vi "EMAPRE_REALTIME_VER2.0.vi"() -> ()   [LabVIEW 2015]
uses:
  <vilib>/Platform/TimedLoop/XDataNode/timing_clust.ctl
  <vilib>/Platform/TimedLoop/XDataNode/nitl_modes.ctl
  <vilib>/Platform/TimedLoop/XDataNode/wakeup.ctl
  <vilib>/myRIO/Common/Instrument Driver Framework/myRIO v1.0/AI/vis/myRIO v1.1 Open AI.vi
  <vilib>/myRIO/Common/Instrument Driver Framework/myRIO v1.0/UART/vis/myRIO v1.0 Close UART.vi
  <vilib>/myRIO/Common/Instrument Driver Framework/Utilities/vis/Validate Channels.vi
  <vilib>/myRIO/Common/Instrument Driver Framework/myRIO v1.0/AI/vis/myRIO v1.0 Reserve AI.vi
  <vilib>/myRIO/Common/Instrument Driver Framework/myRIO v1.0/AI/vis/myRIO v1.0 Build MUX Configuration AI.vi
  <vilib>/myRIO/Common/Instrument Driver Framework/myRIO v1.0/Resource Manager/vis/myRIO v1.0 Reserve Channel List.vi
  <vilib>/myRIO/Common/Instrument Driver Framework/myRIO v1.0/Resource Manager/vis/myRIO v1.0 Reserve Channel.vi
  <vilib>/myRIO/Common/Instrument Driver Framework/myRIO v1.0/Resource Manager/vis/myRIO v1.0 Unreserve Channel.vi
  <vilib>/myRIO/Common/Instrument Driver Framework/myRIO v1.0/Resource Manager/vis/myRIO v1.0 Build Mutex Name.vi
  <vilib>/Utility/VariantDataType/GetNumericInfo.vi
  <vilib>/Utility/error.llb/Error Cluster From Error Code.vi
  <vilib>/myRIO/Common/Instrument Driver Framework/myRIO v1.0/myRIO v1.1 Open.vi
  <vilib>/myRIO/Common/Instrument Driver Framework/myRIO v1.0/AI/vis/myRIO v1.0 Get Scaling Constants AI.vi
  <vilib>/myRIO/Common/Instrument Driver Framework/Utilities/vis/IO Manager.vi
  <vilib>/myRIO/Common/Instrument Driver Framework/Utilities/vis/Configuration Manager.vi
  <vilib>/myRIO/Common/Instrument Driver Framework/myRIO v1.0/myRIO v1.0 Close.vi
  <vilib>/myRIO/Common/Instrument Driver Framework/myRIO v1.0/AI/vis/myRIO v1.0 Read AI.vi
  <vilib>/myRIO/Common/Instrument Driver Framework/Utilities/vis/FPGA Ref Manager.vi
  <vilib>/myRIO/Common/Instrument Driver Framework/myRIO v1.0/myRIO v1.0 Reset FPGA.vi
  <vilib>/myRIO/Common/Instrument Driver Framework/myRIO v1.0/IRQ/vis/myRIO v1.0 IRQ Info FGV.vi
  <vilib>/myRIO/Common/Instrument Driver Framework/myRIO v1.0/IRQ/vis/myRIO v1.0 Timer IRQ Info FGV.vi
  <vilib>/myRIO/Common/Instrument Driver Framework/myRIO v1.0/IRQ/vis/myRIO v1.0 ISR Agent.vi
  <vilib>/platform/TimedLoop/XDataNode/XDataNode.xnode
  <vilib>/myRIO/Instrument Drivers/Onboard IO/AI/AI.lvlib
  <vilib>/myRIO/Instrument Drivers/Utilities/Utilities.lvlib
  <vilib>/Platform/TimedLoop/XDataNode/XDNodeRunTimeDep.lvlib
panel:
  in  "Body":string
  in  "Subject":string
  in  "Password":string
  in  "Email":string
  out "Time":timestamp format="%<%H:%M\n%d/%m/%y>T"
  out "Temperature":dbl(graph)
  out "Start Detection":bool
  in  "Current Sensor\nChannel":tag="B/AI0"
  in  "stop 2":bool
  out "Current Signal":dbl(graph)
  out "Fault":bool
  out "Good Condition":bool
  out "Temperature":dbl(slide) scale=0.0..100.0
  out "Temperature\n(Celcius)":dbl
  in  "stop":bool
  in  "Temperature Sensor\nChannel":tag="B/AI0"
  # "Stator Faults Detection on Induction Motor\n based on Electric Signals Measurement"
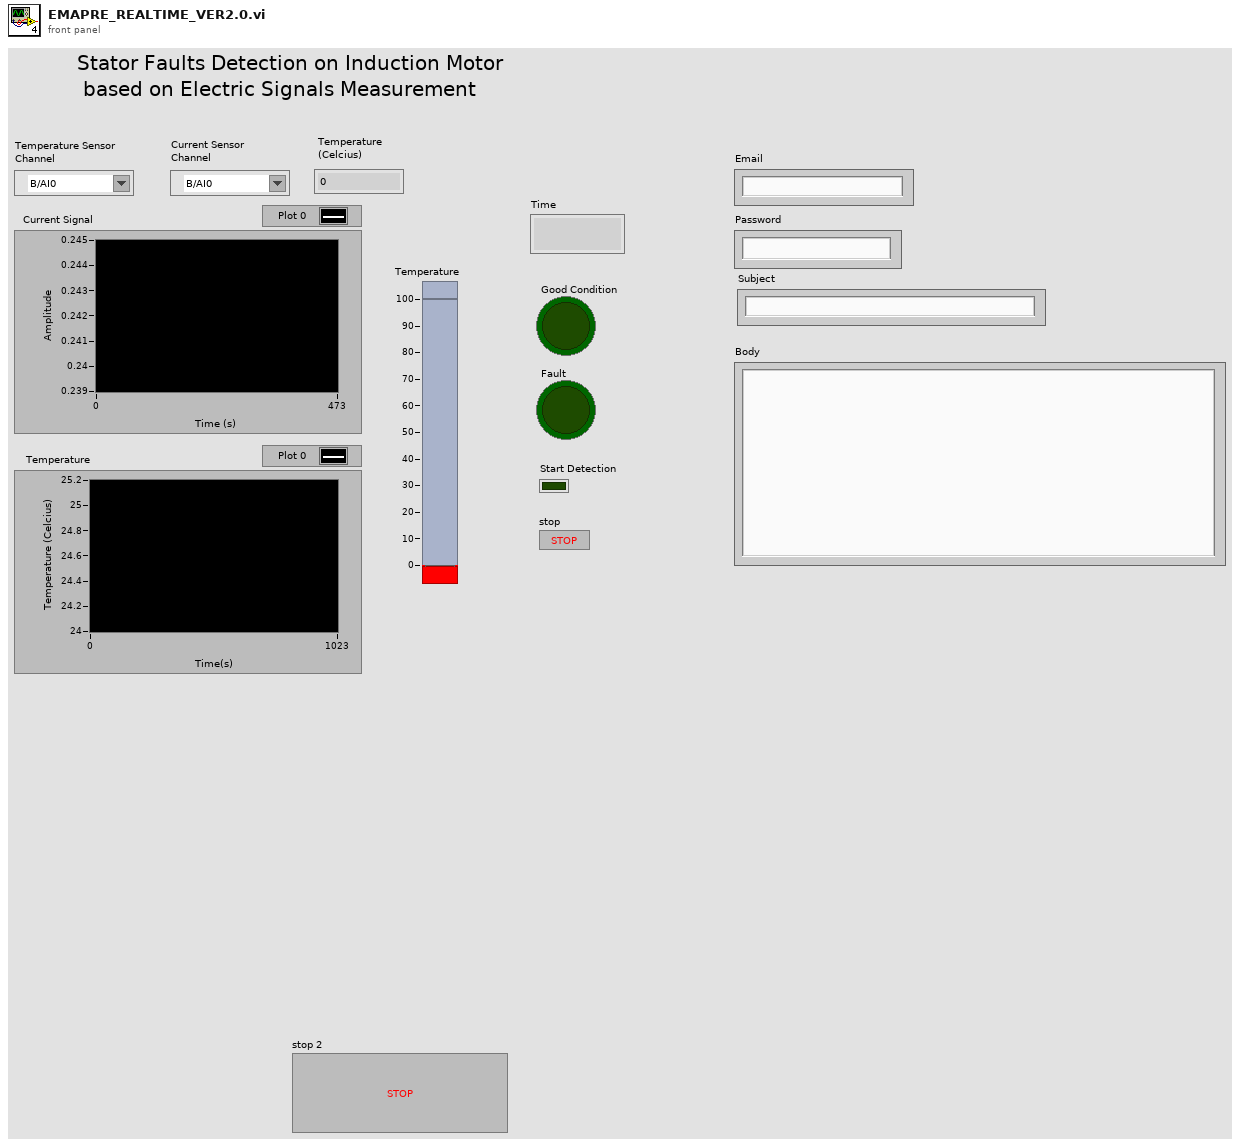
[diagram p1: front panel]
types:
  T1 = typedef "AI.lvlib/AI Reference.ctl" = cluster{"myRIO Reference":T2, "AI Channels List":T6, "AI Scaling Constants List":T8}
  T2 = typedef "myRIO Generic Hardware Reference.ctl" = cluster{"myRIO Model":T3, "myRIO Hardware Reference":T4}
  T3 = typedef "Hardware Version Enum.ctl" = enum16{"Unknown", "myRIO-1900", "myRIO-1950", "roboRIO"}
  T4 = typedef "myRIO v1.0 Reference.ctl" = cluster{"Generic FPGA Reference":T5, "Allow multiple opens":bool}
  T5 = typedef "Generic FPGA Reference.ctl" = refnum<k20>
  T6 = typedef "AI Channels List.ctl" = T7[]
  T7 = typedef "AI Channels Enum.ctl" = enum16{"Not Connected", "AudioIn/Left", "AudioIn/Right", "C/AI0", "C/AI1", "A/AI0", "A/AI1", "A/AI2", "A/AI3", "B/AI0", "B/AI1", "B/AI2", "B/AI3", "AI/AI0", "AI/AI1", "AI/AI2", "AI/AI3"}
  T8 = typedef "Analog Scaling Constants List.ctl" = T9[]
  T9 = typedef "Analog Scaling Constants.ctl" = cluster{"LSB Weight (Volts)":dbl, "Offset (Volts)":dbl, "Signed?":bool}
  T10 = typedef "XDNodeRunTimeDep.lvlib/timing_clust.ctl" = cluster{"Expected End [f-1]":u64, "Actual End [f-1]":u64, "Finished Late? [f-1]":bool, "Expected End [i-1]":u64, "Actual End [i-1]":u64, "Finished Late? [i-1]":bool, "Expected Start [i]":u64, "Actual Start [i]":u64, "Expected Start [f]":u64, "Actual Start [f]":u64, "Source Name":string, "Structure Name":string, "Period":i64, "Deadline":i64, "Offset":i64, "Start":i64, "Priority":i32, "Timeout":i32, "Mode":T11, "Wakeup Reason":T12, "Error":errorcluster, "Source Type":string, "Secondary Source Type":string, "Global End Time":u64, "Global Start Time":u64, "Frame Duration":u64, "Iteration Duration":u64, "Assigned CPU":i32, "I/O Scan Engine Mode":u32}
  T11 = typedef "XDNodeRunTimeDep.lvlib/nitl_modes.ctl" = enum32{"No Change", "Process missed periods, maintain original phase", "Discard missed periods, maintain original phase", "Process missed periods, ignore original phase", "Discard missed periods, ignore original phase"}
  T12 = typedef "XDNodeRunTimeDep.lvlib/wakeup.ctl" = enum32{"Normal", "Aborted", "Asynchronous wakeup", "Timing source error", "Timed loop error", "Timeout"}
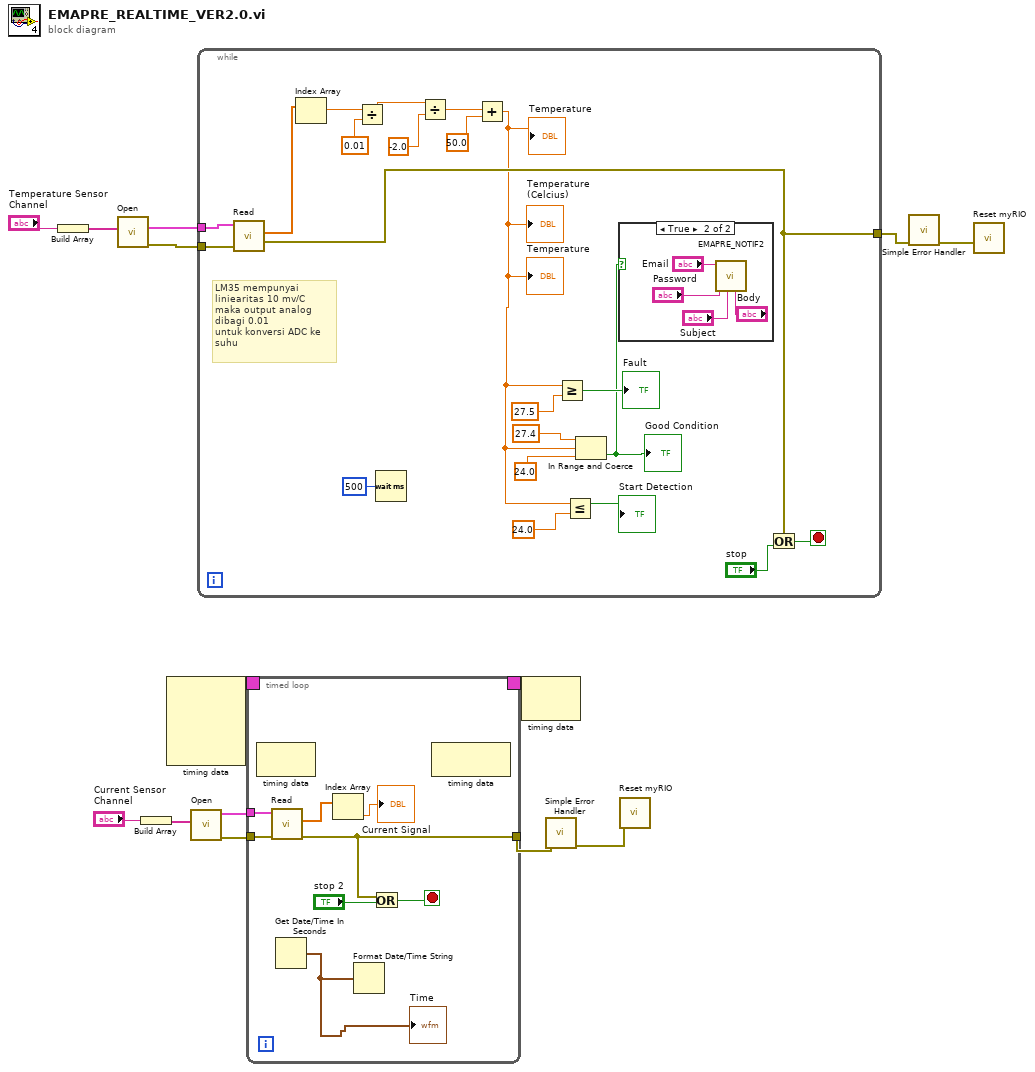
[diagram p0: block diagram]
diagram:
  n1 = Build Array("Temperature Sensor\nChannel") -> (w13:tag[])
  n2 = call <vilib>:"Open.vi"("Channel Names"=w13) -> ("error out"=w4:errorcluster, "AI Ref Out"=w11:T1)  [unwired: 9 in]
  n3 = Build Array("Current Sensor\nChannel") -> (w1:tag[])
  n4 = node-c288() -> (w9:T10)  [unwired: 4 in]
  n5 = call <vilib>:"Open.vi"("Channel Names"=w1) -> ("error out"=w2:errorcluster, "AI Ref Out"=w3:T1)  [unwired: 9 in]
  n6 = while {
    tunnel: w11 -> [w34]
    tunnel: [w31] -> w10
    tunnel: w4 -> [w26]
    stop <- w33 stop-if-true
    # "LM35 mempunyai liniearitas 10 mv/C\nmaka output analog dibagi 0.01\nuntuk konversi ADC ke suhu"
    n7 = call <vilib>:"Read.vi"("error in (no error)"=w26, "AI Ref In"=w34) -> ("error out"=w31:errorcluster, "Values"=w20:dbl[])  [unwired: 7 in, 1 out]
    n8 = Index Array(array=w20) -> (element=w19:dbl)  [unwired: 1 in]
    n9 = Divide(x=w19, y=0.01) -> (x/y=w18:dbl)
    n10 = Wait (ms)(milliseconds to wait=u32 500) -> ()  [unwired: 1 out]
    n11 = Divide(x=w18, y=-2.0) -> (x/y=w24:dbl)
    n12 = Add(x=w24, y=50.0) -> (x+y=w17:dbl)
    "Temperature\n(Celcius)" <- w17
    "Temperature" <- w17
    "Temperature" <- w17
    n13 = Greater Or Equal?(x=w17, y=27.5) -> (x >= y?=→"Fault":bool)
    n14 = Less Or Equal?(x=w17, y=24.0) -> (x <= y?=→"Start Detection":bool)
    n15 = In Range and Coerce(upper limit=27.4, x=w17, lower limit=24.0) -> (In Range?=w15:bool)  [unwired: 1 out]
    "Good Condition" <- w15
    n16 = case shown="True" w15 {
      frame False {
      }
      frame True {
        n17 = call "EMAPRE_NOTIF2.vi"("Body"="Body", "Subject"="Subject", "Password"="Password", "Email"="Email") -> ()  [unwired: 8 in]
      }
    }
    n18 = Or(x=w31, y="stop") -> (x .or. y?=w33:bool)
  }
  n19 = timed-loop {
    timing: w9 -> [_]
    timing-out: [_] -> w8
    tunnel: [w41] -> w5
    tunnel: w3 -> [w43]
    tunnel: w2 -> [w42]
    stop <- w45 stop-if-true
    n20 = node-c288() -> ()  [unwired: 1 in, 1 out]
    n21 = call <vilib>:"Read.vi"("error in (no error)"=w42, "AI Ref In"=w43) -> ("error out"=w41:errorcluster, "Values"=w47:dbl[])  [unwired: 7 in, 1 out]
    n22 = Get Date/Time In Seconds() -> (seconds since 1Jan1904=w40:timestamp)
    "Time" <- w40
    n23 = Index Array(array=w47) -> (element=→"Current Signal":dbl)  [unwired: 1 in]
    n24 = Format Date/Time String(seconds (now)=w40) -> ()  [unwired: 2 in, 1 out]
    n25 = Or(x=w41, y="stop 2") -> (x .or. y?=w45:bool)
    n26 = node-c288() -> ()  [unwired: 1 in, 1 out]
  }
  n27 = node-c288(w8) -> ()  [unwired: 1 out]
  n28 = call <vilib>:"Simple Error Handler.vi"("error in (no error)"=w5) -> ("error out"=w6:errorcluster)  [unwired: 4 in, 4 out]
  n29 = call <vilib>:"Reset myRIO.vi"("error in (no error)"=w6) -> ()  [unwired: 10 in, 1 out]
  n30 = call <vilib>:"Simple Error Handler.vi"("error in (no error)"=w10) -> ("error out"=w12:errorcluster)  [unwired: 4 in, 4 out]
  n31 = call <vilib>:"Reset myRIO.vi"("error in (no error)"=w12) -> ()  [unwired: 10 in, 1 out]
